vi "NotifyIcon - Register LabVIEW User Events.vi"(6 "Action":T1, 8 "error in":errorcluster, 10 "Events to register":T2[](array[typedef]), 11 "NotifyIcon reference in":refnum<k24>) -> (0 "error out":errorcluster, 2 "Event Registration Refnum":refnum<event-registration>, 3 "NotifyIcon reference out":refnum<k24>)   [LabVIEW 2018]
doc: "Registers a LabVIEW user event to allow the LabVIEW Event Structure to capture events fired from the NotifyIcon.\n\nWire the <b>Event Registration Refnum</b> output to the Dynamic Event Terminal of an Event Structure."
uses:
  System.Windows.Forms
  TypeDefs/NotifyIcon Events.ctl
  TypeDefs/NotifyIcon Event Registration Actions.ctl
  TypeDefs/NotifyIcon User Event Ref.ctl
  TypeDefs/NotifyIcon Event Data.ctl
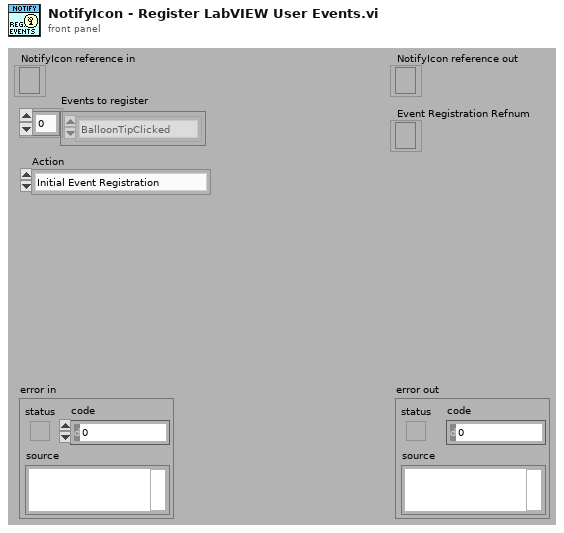
[diagram p1: front panel]
types:
  T1 = typedef "NotifyIcon Event Registration Actions.ctl" = enum16{"Initial Event Registration", "Add to Event Registration", "Destroy Events and Re-register"}
  T2 = typedef "NotifyIcon Events.ctl" = enum16{"BalloonTipClicked", "BalloonTipClosed", "BalloonTipShown", "Click", "Disposed", "DoubleClick", "MouseClick", "MouseDoubleClick", "MouseDown", "MouseMove", "MouseUp", "MenuItemClick", "MenuItemSelect"}
  T3 = typedef "NotifyIcon Event Data.ctl" = cluster{"NotifyIcon Event":T2, "Data String":string}
  T4 = typedef "NotifyIcon User Event Ref.ctl" = refnum<user-event>
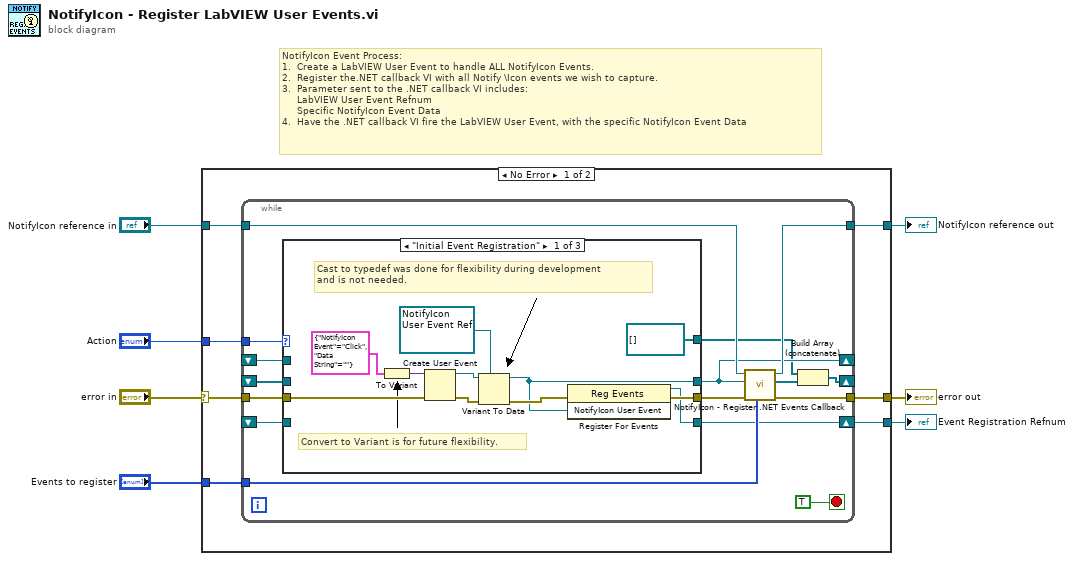
[diagram p0: block diagram]
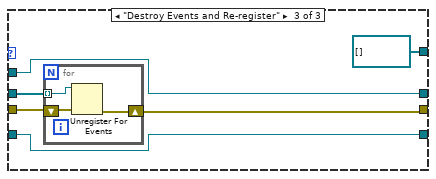
[diagram p3: hidden frame]
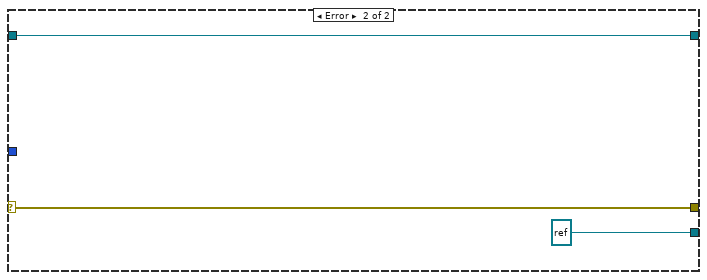
[diagram p4: hidden frame]
diagram:
  # "NotifyIcon Event Process:\n1.  Create a LabVIEW User Event to handle ALL NotifyIcon Events.\n2.  Register the.NET callback VI with all Notify \\Icon events we wish to capture.\n3.  Parameter sent to the .NET callback VI includes:\n     LabVIEW User Event Refnum\n     Specific NotifyIcon Event Data\n4.  Have the .NET callback VI fire the LabVIEW User Event, with the specific NotifyIcon Event Data"
  n1 = case shown="No Error" "error in" {
    selector: "error in" -> [w9 w57]
    tunnel: "NotifyIcon reference in" -> [w14 w55]
    tunnel: "Events to register" -> [w13 _]
    tunnel: [w12 w55] -> w5
    tunnel: [w11 w57] -> w4
    tunnel: [w10 refnum<event-registration> refnum ("Event Registration Refnum")] -> w3
    tunnel: "Action" -> [w8 _]
    frame No Error {
      n2 = while {
        tunnel: w14 -> [w29]
        tunnel: w13 -> [w28]
        tunnel: [w27] -> w12
        tunnel: [w26] -> w11
        tunnel: w9 -> [w24]
        tunnel: w8 -> [w22]
        shift-right: [w21] -> _
        shift-left: _ -> [w20]
        shift-right: [w25] -> w10
        shift-left: _ -> [w19]
        shift-right: [w16] -> _
        shift-left: _ -> [w18]
        stop <- TRUE stop-if-true
        n3 = case shown="\"Initial Event Registration\"" w22 {
          tunnel: [w35 w44 w48] -> w30
          tunnel: [w34 w45 w49] -> w21
          tunnel: [w33 w43 w47] -> w25
          tunnel: w24 -> [w32 w44 w51]
          tunnel: w20 -> [_ w45 w49]
          tunnel: w19 -> [_ w43 w47]
          tunnel: w18 -> [_ w42 w50]
          tunnel: [refnum<k27>[] [] w42 refnum<k27>[] []] -> w15
          frame "Initial Event Registration" {
            # "Cast to typedef was done for flexibility during development\nand is not needed."
            # "Convert to Variant is for future flexibility."
            n4 = To Variant(anything=T3 {"NotifyIcon Event"=enum."Click", "Data String"=""} ("NotifyIcon Event Data")) -> (Variant=w39:variant)
            n5 = Create User Event(user event datatype=w39, error in=w32) -> (user event=w38:refnum<user-event>, error out=w41:errorcluster)
            n6 = Variant To Data(error in=w41, type=T4 refnum ("NotifyIcon User Event"), Variant=w38) -> (data=w34:T4, error out=w40:errorcluster)
            n7 = register-events(error in=w40, w34) -> (reference out=w33:refnum<event-registration>, error out=w35:errorcluster)  [unwired: 1 in]
          }
          frame "Add to Event Registration", Default {
          }
          frame "Destroy Events and Re-register" {
            n8 = for {
              tunnel: w50 -> [w53] mode=indexing
              shift-right: [w52] -> w48
              shift-left: w51 -> [w54]
              n9 = Unregister For Events(event registration refnum=w53, error in=w54) -> (error out=w52:errorcluster)
            }
          }
        }
        n10 = call "NotifyIcon - Register .NET Events Callback.vi"("Events to register"=w28, "error in (no error)"=w30, "NotifyIcon User Event Ref"=w21, "NotifyIcon reference in"=w29) -> ("error out"=w26:errorcluster, ".NET event refs"=w17:refnum<k27>[], "NotifyIcon reference out"=w27:refnum<k24>)  [unwired: 5 in]
        n11 = Build Array (concatenate)(w15, w17) -> (w16:refnum<k27>[])
      }
    }
    frame Error {
    }
  }
  "NotifyIcon reference out" <- w5
  "error out" <- w4
  "Event Registration Refnum" <- w3
